vi "State_Machine.vi"(8 "error in (no error)":errorcluster caption="entrée d'erreur (pas d'erreur)", 11 "Get_Voltage en entrée":refnum<class "Init_SpectumAnalyser.lvclass">) -> (0 "error out":errorcluster caption="sortie d'erreur", 2 "Json_String":string, 3 "Get_Voltage en sortie":refnum<class "Init_SpectumAnalyser.lvclass">)   [LabVIEW 2020, in "Library Test.lvlib" / "Init_SpectumAnalyser.lvclass"]
uses:
  Init_SpectumAnalyser.lvclass
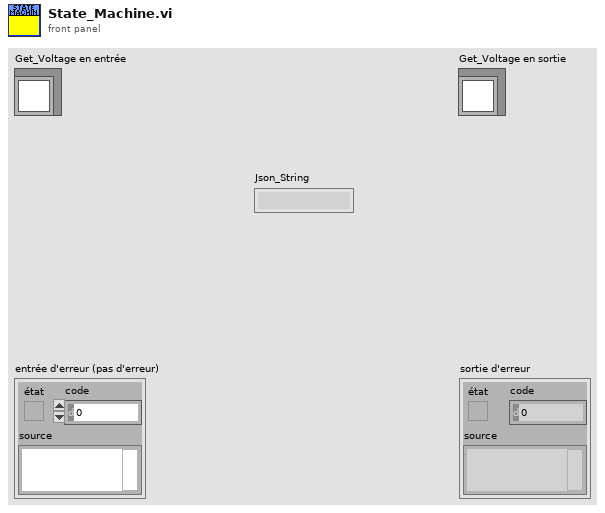
[diagram p1: front panel]
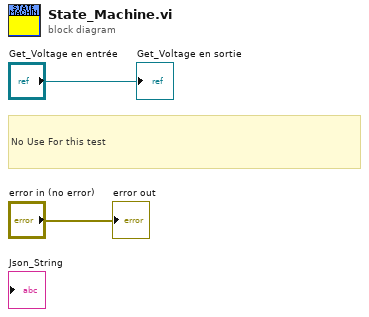
[diagram p0: block diagram]
diagram:
  # "No Use For this test"
  "error out" <- "error in (no error)"
  "Get_Voltage en sortie" <- "Get_Voltage en entrée"
